vi "ep_Zero Crossing Calculation.vi"(5 "dt":dbl, 7 "reset? (F)":bool, 8 "error in (no error)":errorcluster, 9 "group delay":dbl, 10 "parameters":T1, 11 "data in":dbl[](array[numeric])) -> (0 "error out":errorcluster, 2 "average frequency [Hz]":dbl, 3 "zero crossing positions [s]":dbl[](array[numeric]))   [LabVIEW 2013, in "NI_EP_Power Measurement.lvlib"]
uses:
  <vilib>/addons/Electrical Power/Power Measurement/NI_EP_Power Measurement.lvlib
  <vilib>/addons/Electrical Power/PQ/Resampling/Desktop/subVIs/ep_Parameters.ctl
  <vilib>/Analysis/baseanly.llb/Mean (DBL).vi
  <vilib>/addons/Electrical Power/PQ/Resampling/NI_EP_Resample_Host.lvlib
  <vilib>/Analysis/NI_AALBase.lvlib
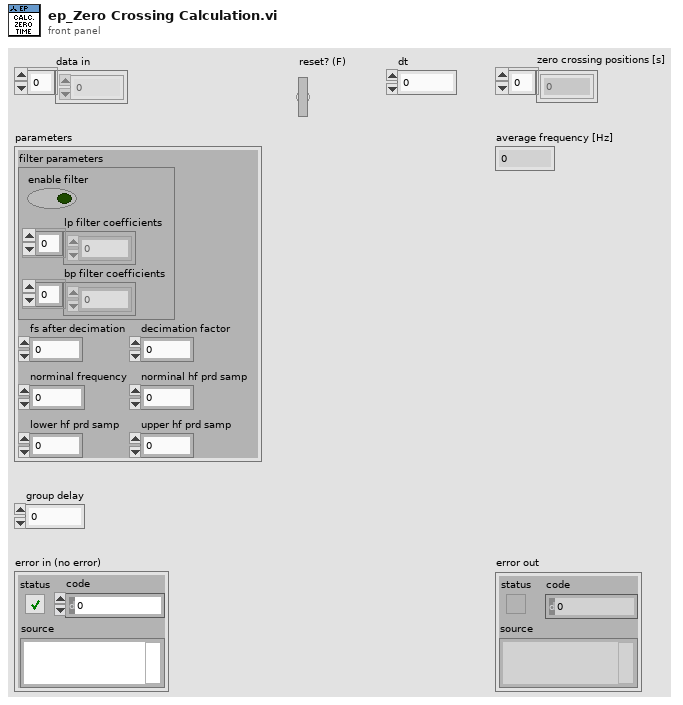
[diagram p1: front panel]
types:
  T1 = typedef "NI_EP_Resample_Host.lvlib/ep_Parameters.ctl" = cluster{"filter parameters":cluster{"enable filter":bool, "lp filter coefficients":dbl[], "bp filter coefficients":dbl[]}, "fs after decimation":dbl, "decimation factor":i32, "norminal frequency":dbl, "norminal hf prd samp":dbl, "lower hf prd samp":i32, "upper hf prd samp":i32}
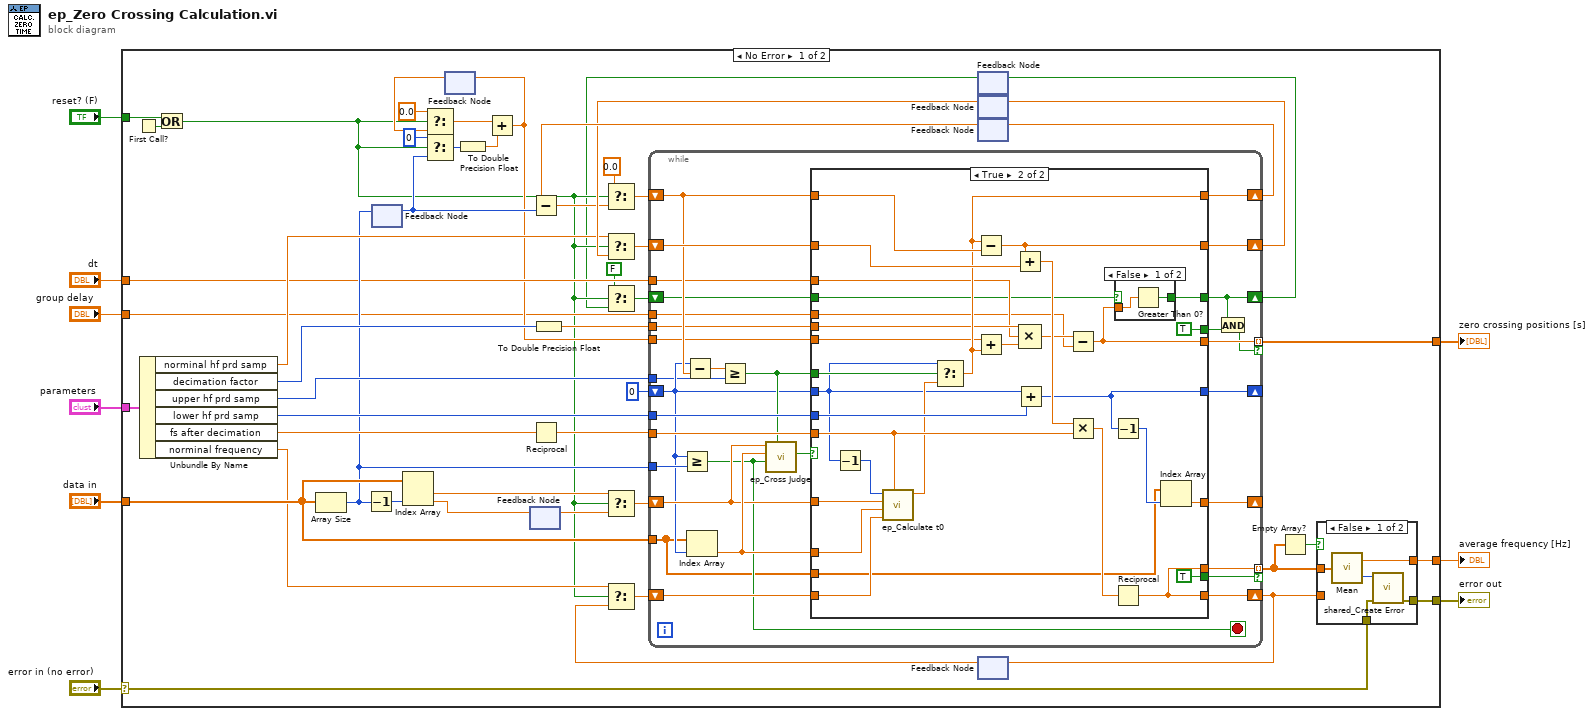
[diagram p0: block diagram]
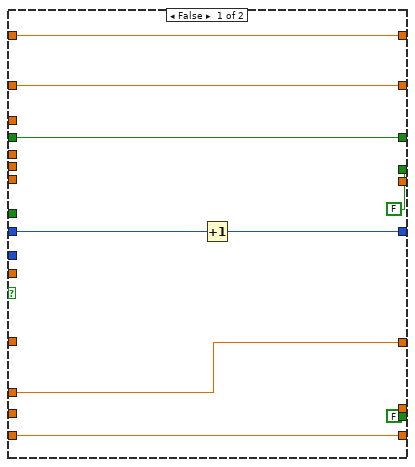
[diagram p3: hidden frame]
diagram:
  n1 = case shown="No Error" "error in (no error)" {
    selector: "error in (no error)" -> [w24 w142]
    tunnel: "data in" -> [w58 _]
    tunnel: [w59 w142] -> w4
    tunnel: "reset? (F)" -> [w60 _]
    tunnel: [w12 _] -> w5
    tunnel: [w25 _] -> w3
    tunnel: "parameters" -> [w26 _]
    tunnel: "dt" -> [w19 _]
    tunnel: "group delay" -> [w16 _]
    frame No Error {
      n2 = First Call?() -> (First Call?: T/F=w47:bool)
      n3 = Unbundle By Name(w26) -> ("norminal hf prd samp"=w32:dbl, "decimation factor"=w31:i32, "upper hf prd samp"=w30:i32, "lower hf prd samp"=w29:i32, "fs after decimation"=w28:dbl, "norminal frequency"=w27:dbl)
      n4 = Or(x=w60, y=w47) -> (x .or. y?=w14:bool)
      n5 = Array Size(array=w58) -> (size(s)=w23:i32)
      n6 = Decrement(x=w23) -> (x-1=w33:i32)
      n7 = feedback #1() -> (w41:i32)  [unwired: 1 in]
      n8 = feedback-in #1(w23) -> ()
      n9 = Index Array(array=w58, index #2=w33) -> (element #1=w52:dbl, element #2=w55:dbl)  [unwired: 1 in]
      n10 = Select(t=0, s=w14, f=w41) -> (s? t:f=w42:i32)
      n11 = feedback #2() -> (w35:dbl)  [unwired: 1 in]
      n12 = Select(t=0.0, s=w14, f=w35) -> (s? t:f=w37:dbl)
      n13 = To Double Precision Float(number=w42) -> (double precision float=w38:dbl)
      n14 = Add(x=w37, y=w38) -> (x+y=w17:dbl)
      n15 = feedback-in #2(w17) -> ()
      n16 = feedback #3() -> (w51:dbl)  [unwired: 1 in]
      n17 = feedback-in #3(w55) -> ()
      n18 = Reciprocal(x=w28) -> (1/x=w39:dbl)
      n19 = To Double Precision Float(number=w31) -> (double precision float=w18:dbl)
      n20 = Select(t=w52, s=w14, f=w51) -> (s? t:f=w50:dbl)
      n21 = feedback #4() -> (w10:bool)  [unwired: 1 in]
      n22 = Select(t=FALSE ("x .or. y?"), s=w14, f=w10) -> (s? t:f=w15:bool)
      n23 = feedback #5() -> (w49:dbl)  [unwired: 1 in]
      n24 = Select(t=w32, s=w14, f=w49) -> (s? t:f=w48:dbl)
      n25 = feedback #6() -> (w56:dbl)  [unwired: 1 in]
      n26 = Subtract(x=w56, y=w41) -> (x-y=w34:dbl)
      n27 = Select(t=0.0, s=w14, f=w34) -> (s? t:f=w46:dbl)
      n28 = feedback #7() -> (w44:dbl)  [unwired: 1 in]
      n29 = Select(t=w27, s=w14, f=w44) -> (s? t:f=w43:dbl)
      n30 = while {
        shift-right: [w82] -> _
        shift-left: w50 -> [w87]
        tunnel: w58 -> [w78]
        shift-right: [w98] -> _
        shift-left: 0 -> [w83]
        shift-right: [w91] -> w54
        shift-left: w46 -> [w84]
        tunnel: w39 -> [w97]
        shift-right: [w96] -> w53
        shift-left: w48 -> [w95]
        shift-right: [w81] -> w20
        shift-left: w43 -> [w94]
        tunnel: w29 -> [w90]
        tunnel: w23 -> [w86]
        tunnel: w30 -> [w77]
        tunnel: [w79] -> w21 mode=indexing if=w80
        tunnel: w19 -> [w76]
        tunnel: w18 -> [w75]
        tunnel: w17 -> [w74]
        tunnel: w16 -> [w73]
        tunnel: [w71] -> w12 mode=indexing if=w69
        shift-right: [w68] -> w11
        shift-left: w15 -> [w72]
        stop <- w85 stop-if-true
        n31 = Greater Or Equal?(x=w83, y=w86) -> (x >= y?=w85:bool)
        n32 = Subtract(x=w83, y=w84) -> (x-y=w89:dbl)
        n33 = Index Array(array=w78, index=w83) -> (element=w93:dbl)
        n34 = Greater Or Equal?(x=w89, y=w77) -> (x >= y?=w88:bool)
        n35 = call <vilib>:"ep_Cross Judge.vi"("over threshold?"=w88, "over index?"=w85, "y2"=w93, "y1"=w87) -> ("cross"=w92:bool)  [unwired: 7 in]
        n36 = case shown="True" w92 {
          tunnel: w83 -> [w107 w125]
          tunnel: [w106 w123] -> w98
          tunnel: w87 -> [_ w134]
          tunnel: w93 -> [w102 w135]
          tunnel: [w105 w117] -> w91
          tunnel: w84 -> [w105 w128]
          tunnel: w97 -> [_ w133]
          tunnel: [w104 w138] -> w96
          tunnel: w95 -> [w104 w137]
          tunnel: [w103 w119] -> w81
          tunnel: w94 -> [w103 w129]
          tunnel: w90 -> [_ w130]
          tunnel: w88 -> [_ w126]
          tunnel: [w102 w124] -> w82
          tunnel: w78 -> [_ w121]
          tunnel: [FALSE TRUE] -> w80
          tunnel: [_ w119] -> w79
          tunnel: [FALSE TRUE] -> w70
          tunnel: w76 -> [_ w113]
          tunnel: w75 -> [_ w114]
          tunnel: w74 -> [_ w116]
          tunnel: w73 -> [_ w111]
          tunnel: w72 -> [w99 w110]
          tunnel: [_ w108] -> w71
          tunnel: [w99 w109] -> w68
          frame False {
            n37 = Increment(x=w107) -> (x+1=w106:i32)
          }
          frame True {
            n38 = Decrement(x=w125) -> (x-1=w131:i32)
            n39 = call <vilib>:"ep_Calculate t0.vi"("dt"=w133, "freq"=w129, "y2"=w135, "y1"=w134, "t1"=w131) -> ("t0"=w127:dbl)  [unwired: 6 in]
            n40 = Select(t=w125, s=w126, f=w127) -> (s? t:f=w117:dbl)
            n41 = Subtract(x=w117, y=w128) -> (x-y=w138:dbl)
            n42 = Add(x=w116, y=w117) -> (x+y=w115:dbl)
            n43 = Add(x=w138, y=w137) -> (x+y=w132:dbl)
            n44 = Add(x=w125, y=w130) -> (x+y=w123:i32)
            n45 = Compound Arithmetic op=MULTIPLY(w114, w113, w115) -> (w112:dbl)
            n46 = Subtract(x=w112, y=w111) -> (x-y=w108:dbl)
            n47 = Multiply(x=w132, y=w133) -> (x*y=w136:dbl)
            n48 = Decrement(x=w123) -> (x-1=w122:i32)
            n49 = Reciprocal(x=w136) -> (1/x=w119:dbl)
            n50 = case shown="False" w110 {
              selector: w110 -> [_ w141]
              tunnel: w108 -> [w139 _]
              tunnel: [w140 w141] -> w109
              frame False {
                n51 = Greater Than 0?(x=w139) -> (x > 0?=w140:bool)
              }
              frame True {
              }
            }
            n52 = Index Array(array=w121, index=w122) -> (element=w124:dbl)
          }
        }
        n53 = And(x=w68, y=w70) -> (x .and. y?=w69:bool)
      }
      n54 = feedback-in #4(w11) -> ()
      n55 = feedback-in #5(w53) -> ()
      n56 = feedback-in #6(w54) -> ()
      n57 = feedback-in #7(w20) -> ()
      n58 = Empty Array?(array=w21) -> (empty?=w22:bool)
      n59 = case shown="False" w22 {
        tunnel: [w65 w66] -> w59
        tunnel: [w63 w67] -> w25
        tunnel: w24 -> [w62 w66]
        tunnel: w21 -> [w61 _]
        tunnel: w20 -> [_ w67]
        frame False {
          n60 = call-poly <vilib>:"Mean.vi"("X"=w61) -> ("mean"=w63:dbl, "error"=w64:i32)
          n61 = call <vilib>:"shared_Create Error.vi"("error in (no error)"=w62, "error code (0)"=w64) -> ("error out"=w65:errorcluster)  [unwired: 9 in]
        }
        frame True {
        }
      }
    }
    frame Error {
    }
  }
  "error out" <- w4
  "zero crossing positions [s]" <- w5
  "average frequency [Hz]" <- w3
